vi "Problem 19 - Counting Sundays.vi"(8 "error in (no error)":errorcluster) -> (0 "error out":errorcluster)   [LabVIEW 2021, in "Project Euler.lvlib"]
uses:
  Project Euler.lvlib
  months_of_the_year enum.ctl
  days_of_the_week enum.ctl
  Utilities/Named Timers/Named Timers.lvlib
  Utilities/Numeric Utilities/Numeric Utilities.lvlib
panel:
  out "current day":i32
  out "current month":T1
  out "current year":u32
  in  "Stop early":bool
  out "Answer = no. of Sundays that fell on the first of the month between 1 Jan 1901 and 31 Dec 2000":i32
  out "Total execution time (ms)":u32
  # "Development\ncontrols/indicators useful for development and testing, but which are not outputs of the VI"
  # "Input\nInputs to the VI"
  # "Output\nOutputs of the VI"
  # "Description\n\nBlank VI with error handling case. \n\nSummarize the use of this VI in this space."
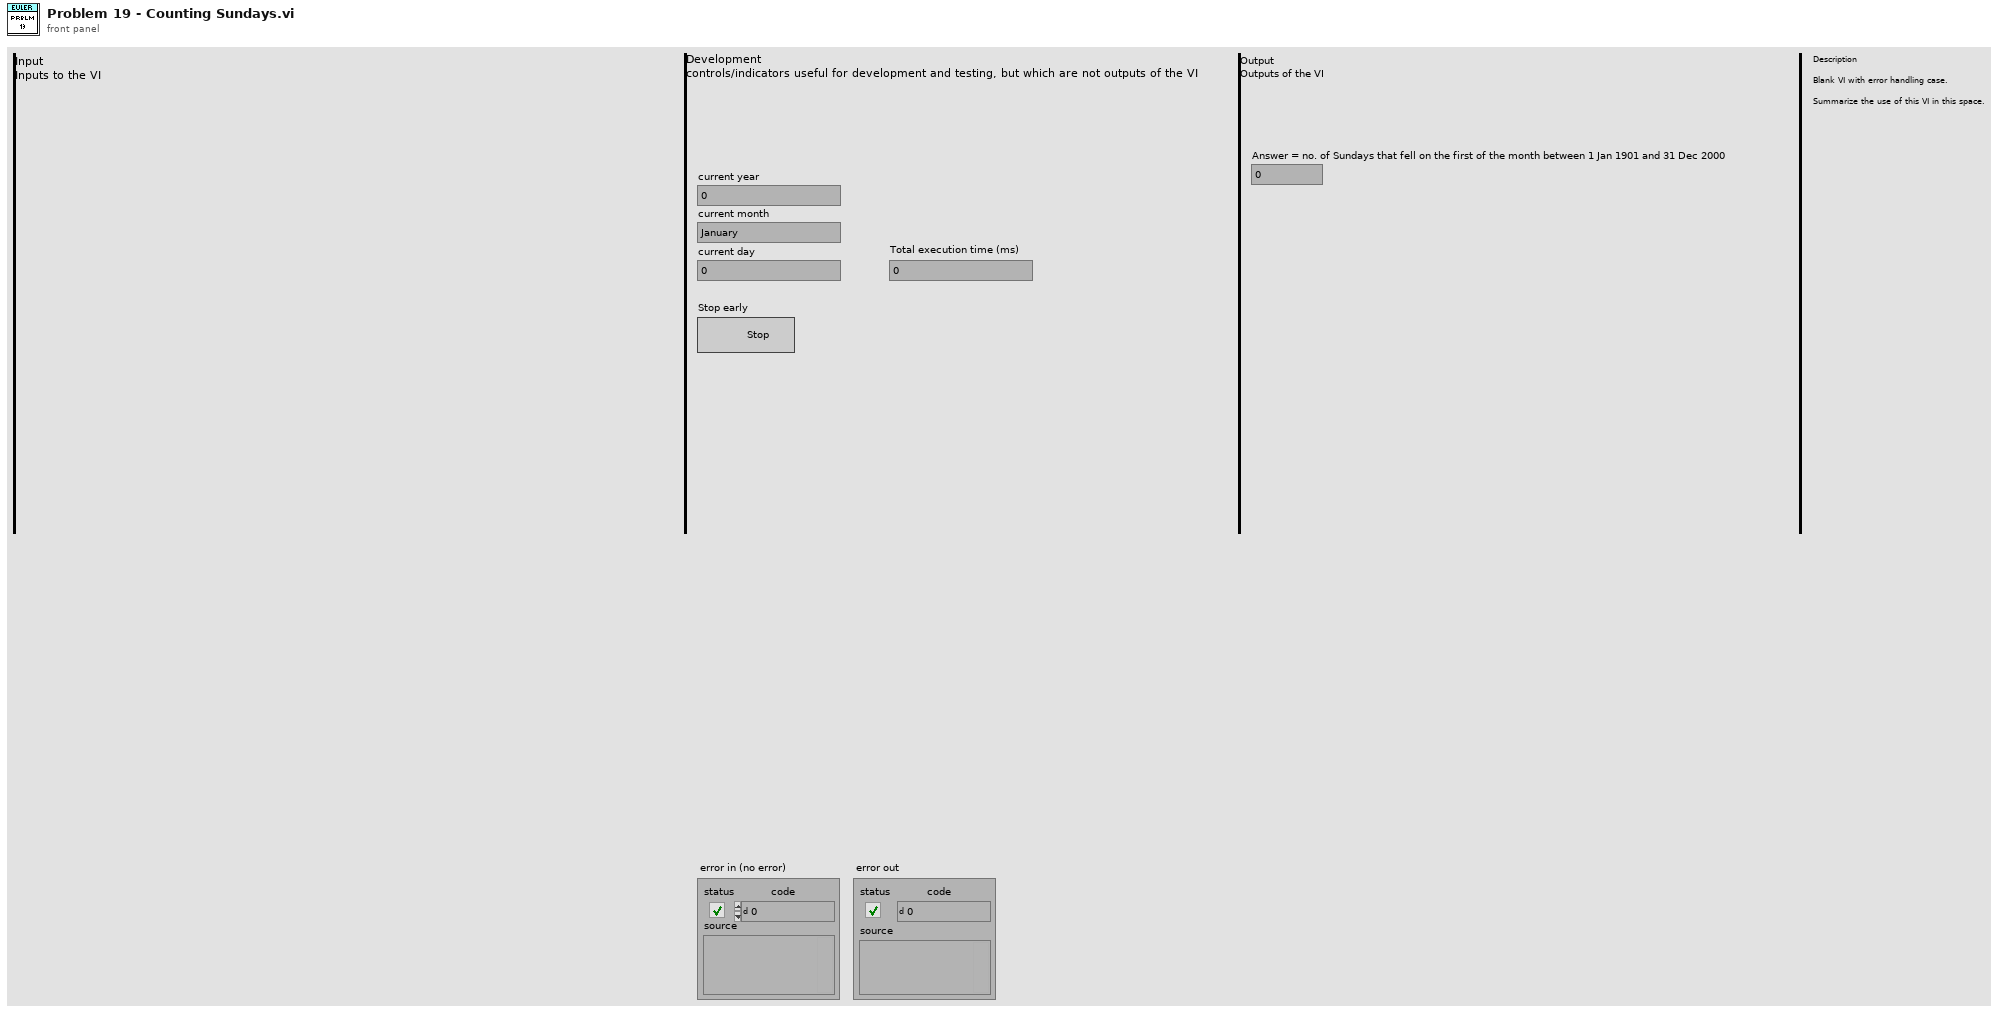
[diagram p1: front panel]
types:
  T1 = typedef "Project Euler.lvlib/months_of_the_year enum.ctl" = enum16{"January", "February", "March", "April", "May", "June", "July", "August", "September", "October", "November", "December"}
  T2 = typedef "Project Euler.lvlib/days_of_the_week enum.ctl" = enum16{"Monday", "Tuesday", "Wednesday", "Thursday", "Friday", "Saturday", "Sunday"}
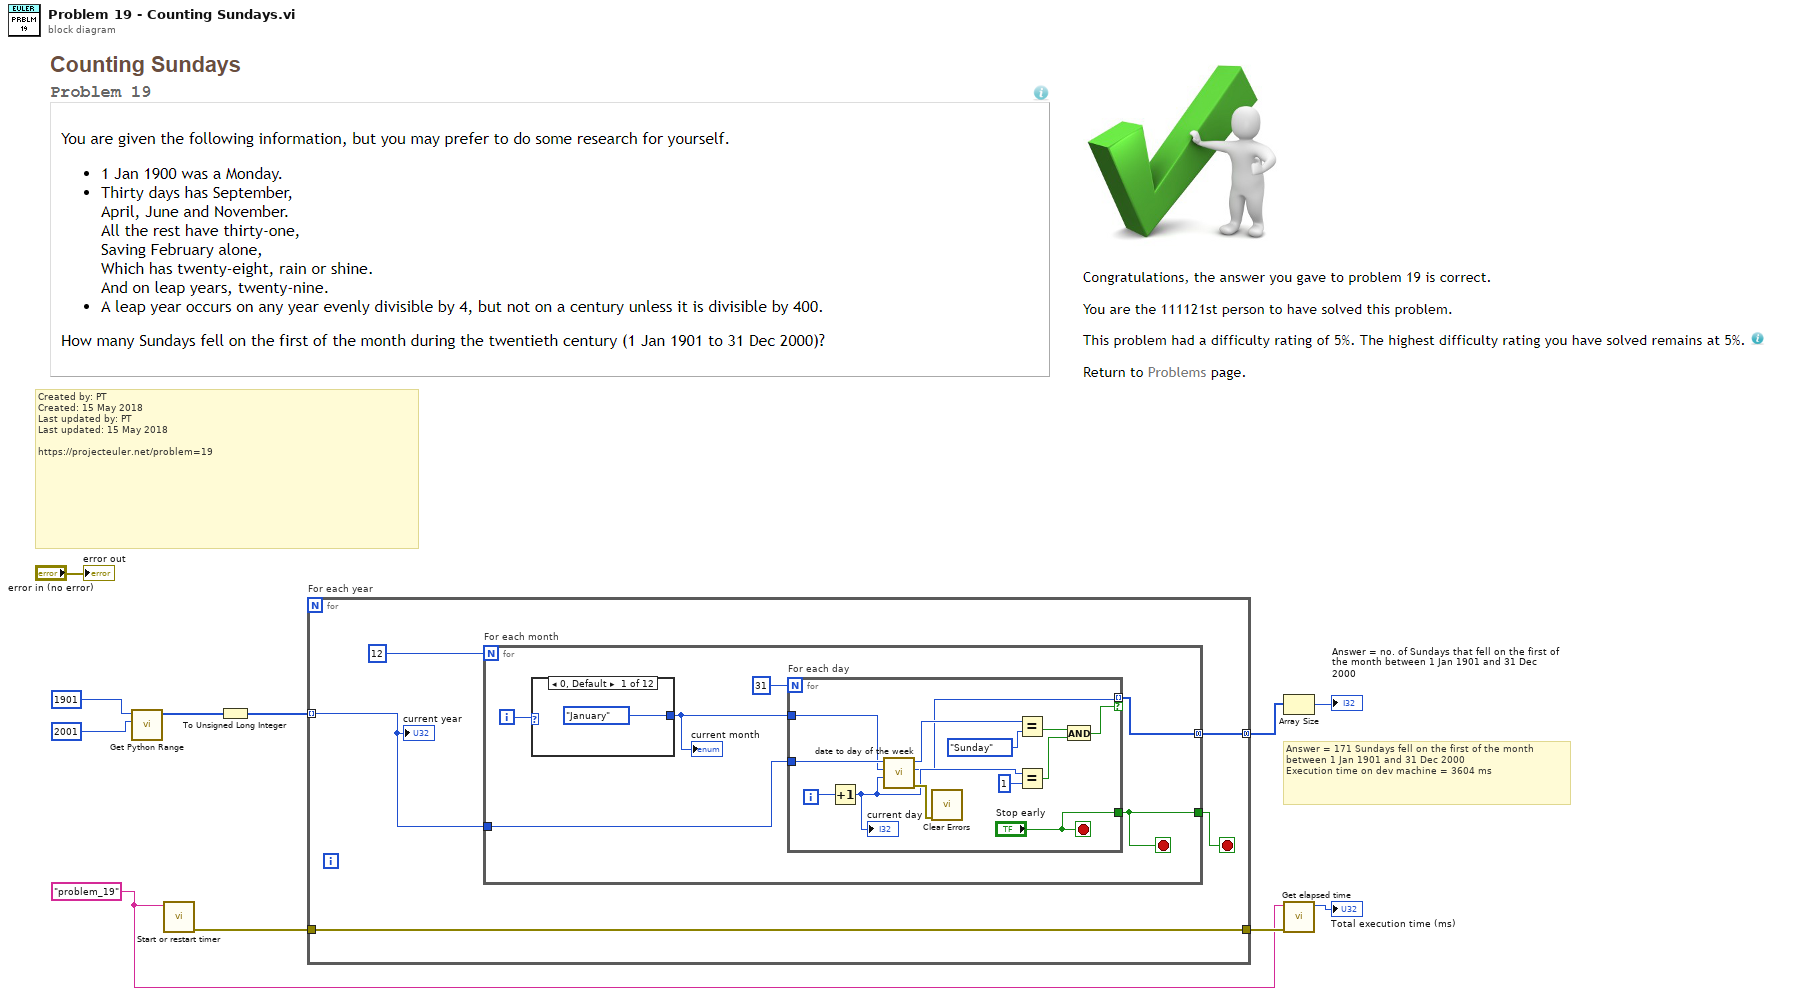
[diagram p0: block diagram]
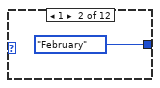
[diagram p2: hidden frame]
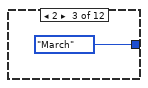
[diagram p3: hidden frame]
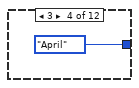
[diagram p4: hidden frame]
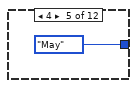
[diagram p5: hidden frame]
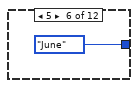
[diagram p6: hidden frame]
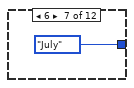
[diagram p7: hidden frame]
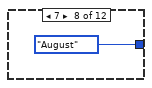
[diagram p8: hidden frame]
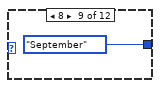
[diagram p9: hidden frame]
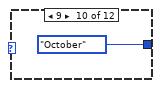
[diagram p10: hidden frame]
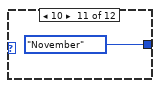
[diagram p11: hidden frame]
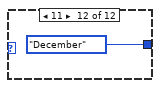
[diagram p12: hidden frame]
diagram:
  w5 = "problem_19" ("Timer name")
  # "Answer = 171 Sundays fell on the first of the month between 1 Jan 1901 and 31 Dec 2000\nExecution time on dev machine = 3604 ms"
  # "Created by: PT\nCreated: 15 May 2018\nLast updated by: PT\nLast updated: 15 May 2018\n\nhttps://projecteuler.net/problem=19"
  n1 = call "Get Python Range.vi"("stop"=u32 2001 ("Year"), "start"=u32 1901 ("Year")) -> ("range"=w2:i32[])  [unwired: 8 in, 1 out]
  n2 = call "Start or restart timer.vi"("Timer name"=w5) -> ("error out"=w7:errorcluster)  [unwired: 10 in]
  n3 = To Unsigned Long Integer(number=w2) -> (unsigned 32bit integer=w1:u32[])
  n4 = for "For each year" {
    tunnel: [w15] -> w9 mode=concatenating
    tunnel: w7 -> [w13]
    tunnel: [w13] -> w6
    tunnel: w1 -> [w12] mode=indexing
    stop <- w14 stop-if-true
    n5 = for "For each month" {
      N: 12 -> [_]
      tunnel: w12 -> [w19]
      tunnel: [w17] -> w15 mode=concatenating
      tunnel: [w18] -> w14
      i -> [w22]
      stop <- w18 stop-if-true
      n6 = case shown="0, Default" w22 {
        tunnel: [months_of_the_year_enum."January" ("Month") months_of_the_year_enum."February" ("Month") months_of_the_year_enum."March" ("Month") months_of_the_year_enum."April" ("Month") months_of_the_year_enum."May" ("Month") months_of_the_year_enum."June" ("Month") months_of_the_year_enum."July" ("Month") months_of_the_year_enum."August" ("Month") months_of_the_year_enum."September" ("Month") months_of_the_year_enum."October" ("Month") months_of_the_year_enum."November" ("Month") months_of_the_year_enum."December" ("Month")] -> w20
        frame 0, Default {
        }
        frame 1 {
        }
        frame 2 {
        }
        frame 3 {
        }
        frame 4 {
        }
        frame 5 {
        }
        frame 6 {
        }
        frame 7 {
        }
        frame 8 {
        }
        frame 9 {
        }
        frame 10 {
        }
        frame 11 {
        }
      }
      "current month" <- w20
      n7 = for "For each day" {
        N: 31 -> [_]
        tunnel: w20 -> [w33]
        tunnel: w19 -> [w34]
        tunnel: ["Stop early"] -> w18
        tunnel: [w24] -> w17 mode=indexing if=w23
        i -> [w32]
        stop <- "Stop early" stop-if-true
        n8 = Increment(x=w32) -> (x+1=w27:i32)
        "current day" <- w27
        n9 = call "date to day of the week.vi"("Day"=w27, "Month"=w33, "Year"=w34) -> ("error out"=w35:errorcluster, "no. of days since 1 Jan 1900"=w24:u32, "Day of the week"=w31:T2)  [unwired: 5 in, 1 out]
        n10 = call <vilib>:"Clear Errors.vi"("error in (no error)"=w35) -> ()  [unwired: 5 in, 2 out]
        n11 = Equal?(x=w31, y=days_of_the_week_enum."Sunday") -> (x = y?=w29:bool)
        n12 = Equal?(x=w27, y=1) -> (x = y?=w28:bool)
        n13 = And(x=w29, y=w28) -> (x .and. y?=w23:bool)
      }
    }
    "current year" <- w12
  }
  n14 = Array Size(array=w9) -> (size(s)=→"Answer = no. of Sundays that fell on the first of the month between 1 Jan 1901 and 31 Dec 2000":i32)
  n15 = call "Get elapsed time.vi"("error in (no error)"=w6, "Timer name"=w5) -> ("Elapsed time (ms)"=→"Total execution time (ms)":u32)  [unwired: 6 in, 3 out]
  "error out" <- "error in (no error)"
